vi "Local_Path_Second (SubVI).vi"(2 "heading_deg":dbl, 3 "heading_limit":dbl=30.0, 4 "y_long":dbl, 5 "x_lat":dbl, 6 "Y_long_path":dbl[](array[numeric]), 7 "X_lat_path":dbl[](array[numeric])) -> (0 "Dist.WP":dbl, 1 "Index(near vehicle)":i32)   [LabVIEW 2024]
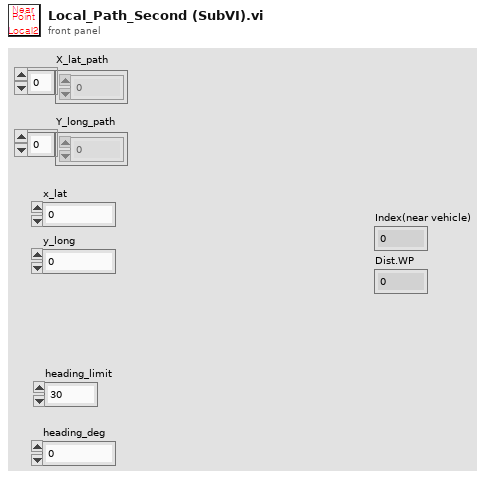
[diagram p1: front panel]
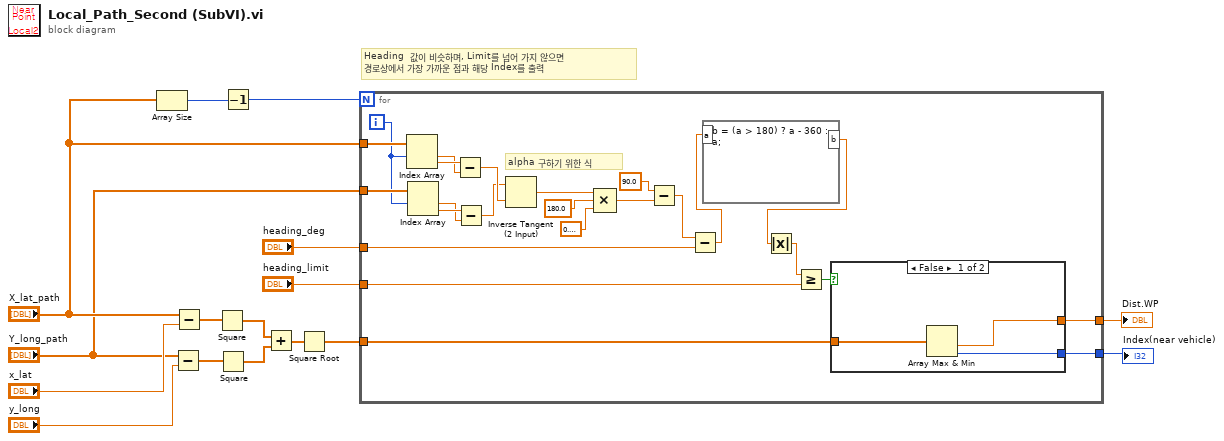
[diagram p0: block diagram]
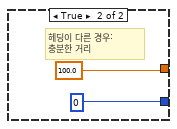
[diagram p2: hidden frame]
diagram:
  # "Heading  값이 비슷하며, Limit를 넘어 가지 않으면\n경로상에서 가장 가까운 점과 해당 Index를 출력"
  n1 = Array Size(array="X_lat_path") -> (size(s)=w9:i32)
  n2 = Subtract(x="Y_long_path", y="y_long") -> (x-y=w13:dbl[])
  n3 = Subtract(x="X_lat_path", y="x_lat") -> (x-y=w15:dbl[])
  n4 = Square(x=w15) -> (x^2=w12:dbl[])
  n5 = Square(x=w13) -> (x^2=w11:dbl[])
  n6 = Decrement(x=w9) -> (x-1=w8:i32)
  n7 = Add(x=w12, y=w11) -> (x+y=w10:dbl[])
  n8 = Square Root(x=w10) -> (sqrt(x)=w3:dbl[])
  n9 = for {
    N: w8 -> [_]
    tunnel: w3 -> [w25]
    tunnel: "X_lat_path" -> [w40]
    tunnel: "Y_long_path" -> [w39]
    tunnel: "heading_deg" -> [w31]
    tunnel: "heading_limit" -> [w29]
    tunnel: [w23] -> w2
    tunnel: [w22] -> w1
    i -> [w28]
    # "alpha 구하기 위한 식"
    n10 = Index Array(array=w40, index #1=w28) -> (element #1=w37:dbl, element #2=w38:dbl)  [unwired: 1 in]
    n11 = Index Array(array=w39, index #1=w28) -> (element #1=w35:dbl, element #2=w36:dbl)  [unwired: 1 in]
    n12 = Subtract(x=w38, y=w37) -> (x-y=w27:dbl)
    n13 = Subtract(x=w36, y=w35) -> (x-y=w26:dbl)
    n14 = Inverse Tangent (2 Input)(1:w27, 2:w26) -> (0:w34:dbl)
    n15 = Compound Arithmetic op=MULTIPLY(w34, 180.0 ("value"), 0.3183098861837907) -> (w21:dbl)
    n16 = Subtract(x=90.0, y=w21) -> (x-y=w19:dbl)
    n17 = Subtract(x=w19, y=w31) -> (x-y=w18:dbl)
    n18 = formula code="b = (a > 180) ? a - 360 : a;"("a"=w18) -> ("b"=w17:dbl)
    n19 = Absolute Value(x=w17) -> (abs(x)=w30:dbl)
    n20 = Greater Or Equal?(x=w30, y=w29) -> (x >= y?=w24:bool)
    n21 = case shown="False" w24 {
      tunnel: w25 -> [w43 _]
      tunnel: [w42 100.0] -> w23
      tunnel: [w41 0] -> w22
      frame False {
        n22 = Array Max & Min(array=w43) -> (min value=w42:dbl, min index (indices)=w41:i32)  [unwired: 2 out]
      }
      frame True {
        # "헤딩이 다른 경우:\n충분한 거리"
      }
    }
  }
  "Dist.WP" <- w2
  "Index(near vehicle)" <- w1
